vi "GetFilesValise.vi"(4 "error in (no error)":errorcluster, 6 "Test Num :":u32, 7 "Project :":string) -> (0 "error out":errorcluster, 3 "NomProjetOut":string)   [LabVIEW 2017]
uses:
  DefDeType/WhichPath.ctl
panel:
  out "Nortek File":bool
  out "Hexapod File":bool
  out "Qualisys file":bool
  out "Valise file":bool
  out "Slide":u8(slide) scale=0.0..10.0
  in  "Etat":string
  # "Downloading files"
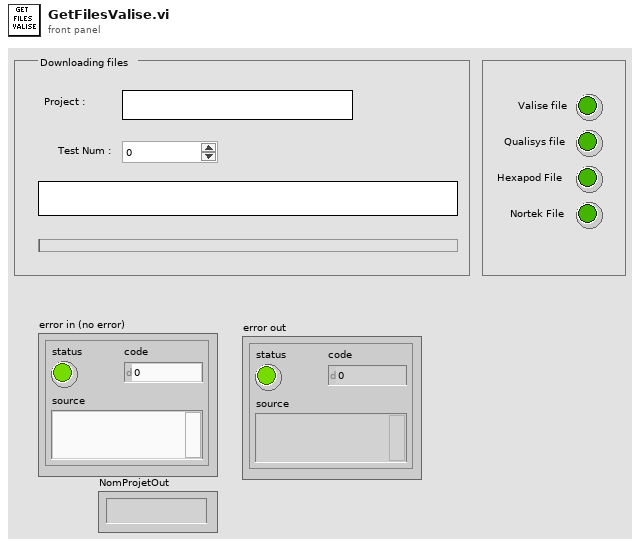
[diagram p1: front panel]
types:
  T1 = typedef "WhichPath.ctl" = enum16{"DossierProjet", "Config", "Meas", "MeasSuitCase", "MeasOnBoard", "MeasQualisys", "MeasTDMS", "MeasHexapode", "MeasNortek", "Fig", "Res", "MeasUSB"}
  T2 = typedef "ConfigTotale.ctl" = cluster{"VoltageChannels":T3, "WheastoneBridgeChannels":T4, "Configuration":T5}
  T3 = typedef "VoltageChannels.ctl" = cluster{"ChannelNames":string[], "Sensitivity(Unit/V)":dbl[], "AutoZero":bool[], "ChannelUnits":string[], "Offsets(Units)":dbl[], "Graph Num":u8[]}
  T4 = typedef "WBridgeChannels.ctl" = cluster{"ChannelNames":string[], "Sensitivity(Unit/V)":dbl[], "AutoZero":bool[], "ChannelUnits":string[], "Offsets(Units)":dbl[], "Graph Num":u8[]}
  T5 = typedef "Configuration.ctl" = cluster{"AcqSamplingRate(Hz)":u32, "AcqTime(s)":u32, "Trigger":bool, "NbVoltageChannels":u32, "NbWBridgeChannels":u32, "Qualisys":bool, "Hexapode":bool, "FinalSamplingRate(Hz)":u32, "QualisysDataType":enum16{"6DOF", "3DTracking", "6DOF + 3D"}, "Nortek":bool, "HBM":bool}
  T6 = typedef "WhichPath.ctl" = enum16{"DossierProjet", "Config", "Meas", "MeasPCI", "MeasCRIO1", "MeasCRIO2", "MeasQualisys", "MeasHBM", "MeasTDMS", "Fig", "Res"}
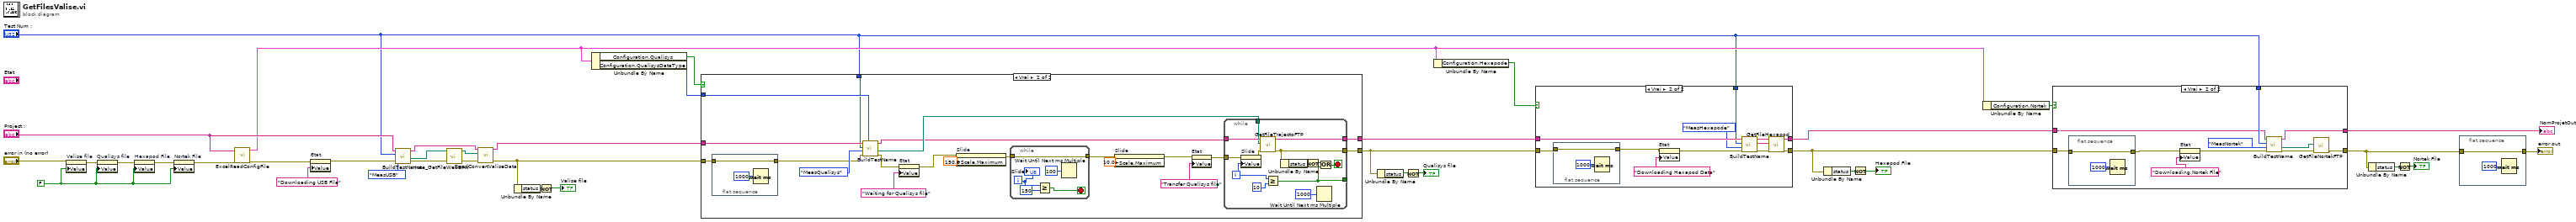
[diagram p0: block diagram]
diagram:
  w26 = FALSE ("Valise file")
  n1 = property on="Valise file" class="Bool (strict)"(error in="error in (no error)", "Value"=w26) -> (error out=w30:errorcluster)  [unwired: 1 in, 1 out]
  n2 = property on="Qualisys file" class="Bool (strict)"(error in=w30, "Value"=w26) -> (error out=w29:errorcluster)  [unwired: 1 in, 1 out]
  n3 = property on="Hexapod File" class="Bool (strict)"(error in=w29, "Value"=w26) -> (error out=w28:errorcluster)  [unwired: 1 in, 1 out]
  n4 = property on="Nortek File" class="Bool (strict)"(error in=w28, "Value"=w26) -> (error out=w27:errorcluster)  [unwired: 1 in, 1 out]
  n5 = call "ExcelReadConfigFile.vi"("NomProjet"="Project :", "error in (no error)"=w27) -> ("ConfigurationTotale"=w15:T2, "error out"=w38:errorcluster)  [unwired: 3 in]
  n6 = property on="Etat" class="Ch"(error in=w38, "Value"="Downloading USB File" ("Etat")) -> (error out=w35:errorcluster)  [unwired: 1 in, 1 out]
  n7 = call "BuildTestName.vi"("entrée d'erreur"=w35, "WhichPath?"=WhichPath."MeasUSB", "NextTestNum"="Test Num :", "NomProjet"="Project :") -> ("sortie d'erreur"=w36:errorcluster, "cheminProchainFichier"=w37:path, "NomProjetOut"=w5:string)  [unwired: 1 in, 1 out]
  n8 = call "Hote_GetFileWebDAV.vi"("error in"=w36, "NewValiseFile"=w37) -> ("error out"=w7:errorcluster, "NewValiseFileOUT"=w6:path)  [unwired: 2 in]
  n9 = call "ReadConvertValiseData.vi"("entrée d'erreur"=w7, "ValiseFileIN"=w6, "NomProjet"=w5) -> ("sortie d'erreur"=w1:errorcluster, "ProjetOUT"=w4:string)  [unwired: 2 in, 1 out]
  n10 = Unbundle By Name(w1) -> ("status"=w32:bool)
  n11 = Not(x=w32) -> (.not. x?=→"Valise file":bool)
  n12 = Unbundle By Name(w15) -> ("Configuration.Qualisys"=w24:bool, "Configuration.QualisysDataType"=w23:enum16{"6DOF", "3DTracking", "6DOF + 3D"})
  n13 = case shown="Vrai" w24 {
    tunnel: w1 -> [w41 w43]
    tunnel: w4 -> [w40 w48]
    tunnel: w23 -> [_ w47]
    tunnel: "Test Num :" -> [_ w46]
    tunnel: [w41 w45] -> w3
    tunnel: [w40 w44] -> w20
    frame False {
    }
    frame True {
      n14 = flat-sequence {
        tunnel: w43 -> [w63]
        tunnel: [w63] -> w42
        frame #0 {
          n15 = Wait (ms)(milliseconds to wait=u32 1000) -> ()  [unwired: 1 out]
        }
      }
      n16 = call "BuildTestName.vi"("QualisysDataType"=w47, "entrée d'erreur"=w42, "WhichPath?"=WhichPath."MeasQualisys", "NextTestNum"=w46, "NomProjet"=w48) -> ("sortie d'erreur"=w49:errorcluster, "cheminProchainFichier"=w61:path, "NomProjetOut"=w52:string)  [unwired: 1 out]
      n17 = property on="Etat" class="Ch"(error in=w49, "Value"="Waiting for Qualisys file" ("Etat")) -> (error out=w60:errorcluster)  [unwired: 1 in, 1 out]
      n18 = property on="Slide" class="Gliss (strict)"(error in=w60, "Scale.Maximum"=150.0 ("Scale.Range:Maximum")) -> (error out=w59:errorcluster)  [unwired: 1 in, 1 out]
      n19 = while {
        tunnel: w59 -> [w81]
        tunnel: [w81] -> w55
        i -> [w77]
        stop <- w78 stop-if-true
        n20 = Greater Or Equal?(x=w77, y=150) -> (x >= y?=w78:bool)
        n21 = Wait Until Next ms Multiple(millisecond multiple=u32 100) -> ()  [unwired: 1 out]
        "Slide" <- w77
      }
      n22 = property on="Slide" class="Gliss (strict)"(error in=w55, "Scale.Maximum"=10.0 ("Scale.Range:Maximum")) -> (error out=w56:errorcluster)  [unwired: 1 in, 1 out]
      n23 = property on="Etat" class="Ch"(error in=w56, "Value"="Transfer Qualisys file" ("Etat")) -> (error out=w54:errorcluster)  [unwired: 1 in, 1 out]
      n24 = while {
        tunnel: w52 -> [w71]
        tunnel: w54 -> [w68]
        tunnel: [w70] -> w44
        tunnel: [w69] -> w45
        tunnel: [w72] -> _
        tunnel: w61 -> [w64]
        i -> [w65]
        stop <- w73 stop-if-true
        n25 = property on="Slide" class="Gliss (strict)"(error in=w68, "Value"=w65) -> (error out=w67:errorcluster)  [unwired: 1 in, 1 out]
        n26 = call "GetFileTrajectoFTP.vi"("error in (no error)"=w67, "NewTrajectoFile"=w64, "NomProjet"=w71) -> ("error out"=w69:errorcluster, "NomProjetOut"=w70:string)  [unwired: 3 in]
        n27 = Greater Or Equal?(x=w65, y=10 ("x")) -> (x >= y?=w72:bool)
        n28 = Unbundle By Name(w69) -> ("status"=w75:bool)
        n29 = Not(x=w75) -> (.not. x?=w74:bool)
        n30 = Wait Until Next ms Multiple(millisecond multiple=u32 1000 ("n millisecondes")) -> ()  [unwired: 1 out]
        n31 = Or(x=w74, y=w72) -> (x .or. y?=w73:bool)
      }
    }
  }
  n32 = Unbundle By Name(w3) -> ("status"=w22:bool)
  n33 = Not(x=w22) -> (.not. x?=→"Qualisys file":bool)
  n34 = Unbundle By Name(w15) -> ("Configuration.Hexapode"=w19:bool)
  n35 = case shown="Vrai" w19 {
    tunnel: w3 -> [w83 w85]
    tunnel: [w83 w87] -> w2
    tunnel: [w82 w90] -> w14
    tunnel: w20 -> [w82 w94]
    tunnel: "Test Num :" -> [_ w86]
    frame False {
    }
    frame True {
      n36 = flat-sequence {
        tunnel: w85 -> [w97]
        tunnel: [w97] -> w84
        frame #0 {
          n37 = Wait (ms)(milliseconds to wait=u32 1000) -> ()  [unwired: 1 out]
        }
      }
      n38 = property on="Etat" class="Ch"(error in=w84, "Value"="Downloading Hexapod Data" ("Etat")) -> (error out=w88:errorcluster)  [unwired: 1 in, 1 out]
      n39 = call "BuildTestName.vi"("entrée d'erreur"=w88, "WhichPath?"=WhichPath."MeasHexapode", "NextTestNum"=w86, "NomProjet"=w94) -> ("sortie d'erreur"=w95:errorcluster, "NomProchainFichier"=w91:string, "NomProjetOut"=w92:string)  [unwired: 1 in, 1 out]
      n40 = call "GetFileHexapod.vi"("error in"=w95, "HexpodFileName"=w91, "Projet"=w92) -> ("error out"=w87:errorcluster, "ProjetOut"=w90:string)  [unwired: 2 in, 1 out]
    }
  }
  n41 = Unbundle By Name(w2) -> ("status"=w18:bool)
  n42 = Not(x=w18) -> (.not. x?=→"Hexapod File":bool)
  n43 = Unbundle By Name(w15) -> ("Configuration.Nortek"=w16:bool)
  n44 = case shown="Vrai" w16 {
    tunnel: w2 -> [w98 w101]
    tunnel: [w99 w103] -> w11
    tunnel: w14 -> [w99 w109]
    tunnel: "Test Num :" -> [_ w110]
    tunnel: [w98 w102] -> w9
    frame False {
    }
    frame True {
      n45 = flat-sequence {
        tunnel: w101 -> [w112]
        tunnel: [w112] -> w100
        frame #0 {
          n46 = Wait (ms)(milliseconds to wait=u32 1000) -> ()  [unwired: 1 out]
        }
      }
      n47 = property on="Etat" class="Ch"(error in=w100, "Value"="Downloading Nortek File" ("Etat")) -> (error out=w106:errorcluster)  [unwired: 1 in, 1 out]
      n48 = call "BuildTestName.vi"("entrée d'erreur"=w106, "WhichPath?"=WhichPath."MeasNortek", "NextTestNum"=w110, "NomProjet"=w109) -> ("sortie d'erreur"=w105:errorcluster, "cheminProchainFichier"=w104:path, "NomProjetOut"=w103:string)  [unwired: 1 in, 1 out]
      n49 = call "GetFileNortekFTP.vi"("error in (no error)"=w105, "NewNortekFile"=w104) -> ("error out"=w102:errorcluster)  [unwired: 4 in, 1 out]
    }
  }
  "NomProjetOut" <- w11
  n50 = Unbundle By Name(w9) -> ("status"=w12:bool)
  n51 = Not(x=w12) -> (.not. x?=→"Nortek File":bool)
  n52 = flat-sequence {
    tunnel: w9 -> [w114]
    tunnel: [w114] -> w8
    frame #0 {
      n53 = Wait (ms)(milliseconds to wait=u32 1000) -> ()  [unwired: 1 out]
    }
  }
  "error out" <- w8
